vi "Rcvd Bin Packet.vi"(8 "error in (no error)":errorcluster) -> (0 "error out":errorcluster, 2 "length":u32, 3 "Buff":u8[](array[numeric]))   [LabVIEW 2015, in "TPVG_DLL.lvlib"]
doc: "This function check incomming bytes to found new packet\n\n--------------------------------------------------------------------\nWritten by: Dang Lam"
uses:
  TPVG_DLL.lvlib
  TPVG_DLL.dll
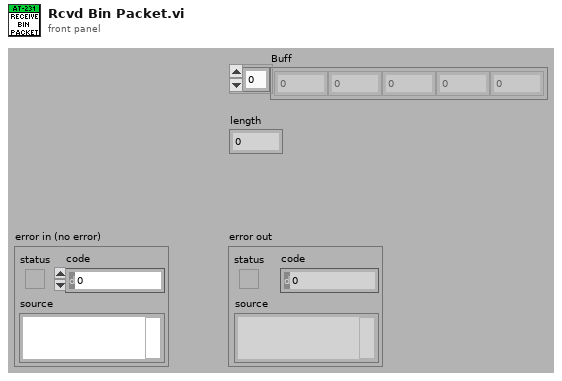
[diagram p1: front panel]
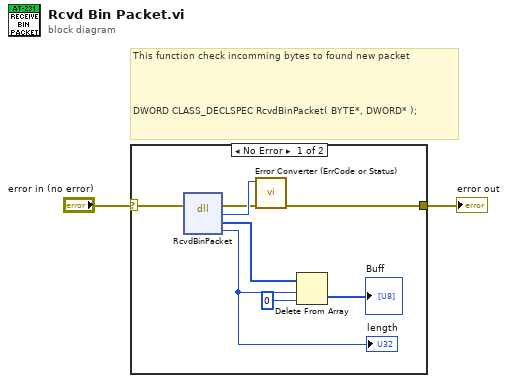
[diagram p0: block diagram]
diagram:
  # "This function check incomming bytes to found new packet\n\n\n\n\nDWORD CLASS_DECLSPEC RcvdBinPacket( BYTE*, DWORD* );"
  n1 = case shown="No Error" "error in (no error)" {
    selector: "error in (no error)" -> [w7 w11]
    tunnel: [w8 w11] -> w2
    frame No Error {
      n2 = dll-call lib="\\\\Mac\\Home/Desktop/imt_test_app 28-06-2012/TPVG_DLL.dll" fn="RcvdBinPacket"(error in=w7) -> (error out=w9:errorcluster, "return type"=w10:u32, "Buff"=w6:u8[], "length"=w5:u32)  [unwired: 4 in, 1 out]
      "length" <- w5
      n3 = call "Error Converter (ErrCode or Status).vi"("error in (no error)"=w9, "error code"=w10) -> ("error out"=w8:errorcluster)  [unwired: 9 in]
      n4 = Delete From Array(array=w6, length=w5, index=0) -> (deleted portion=→"Buff":u8[])  [unwired: 1 out]
    }
    frame Error {
    }
  }
  "error out" <- w2
